vi "HandlePostRequest.vi"(12 "LabVIEW Web Service Request":refnum<class "Web Request.lvclass">) -> (1 "Open %":dbl, 2 "Status":string, 13 "Message":string)   [LabVIEW 2024]
uses:
  <vilib>/wsapi/Web Request.lvclass
  D/Global.vi
  <vilib>/Instr/_visa.llb/VISA Configure Serial Port (Instr).vi
panel:
  out "usb out 2":string
  out "usb out":string
  # "Use the Web Service Request input terminal to call the VIs on the Web Services palette. Do not remove it from the connector pane unless you don't need access to the palette."
  # "Each additional control wired to the connector pane will be available as an input in the URL. To include an indicator in terminal-mode output (the default setting), it must also be wired to the connector pane."
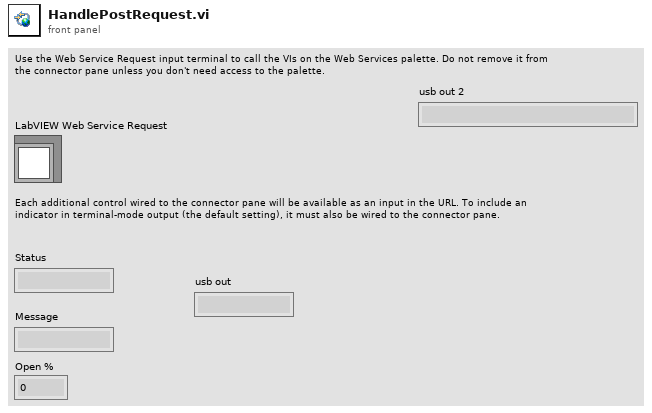
[diagram p1: front panel]
types:
  T1 = cluster{"mode":string, "value":dbl, "t_open":dbl, "t_close":dbl}
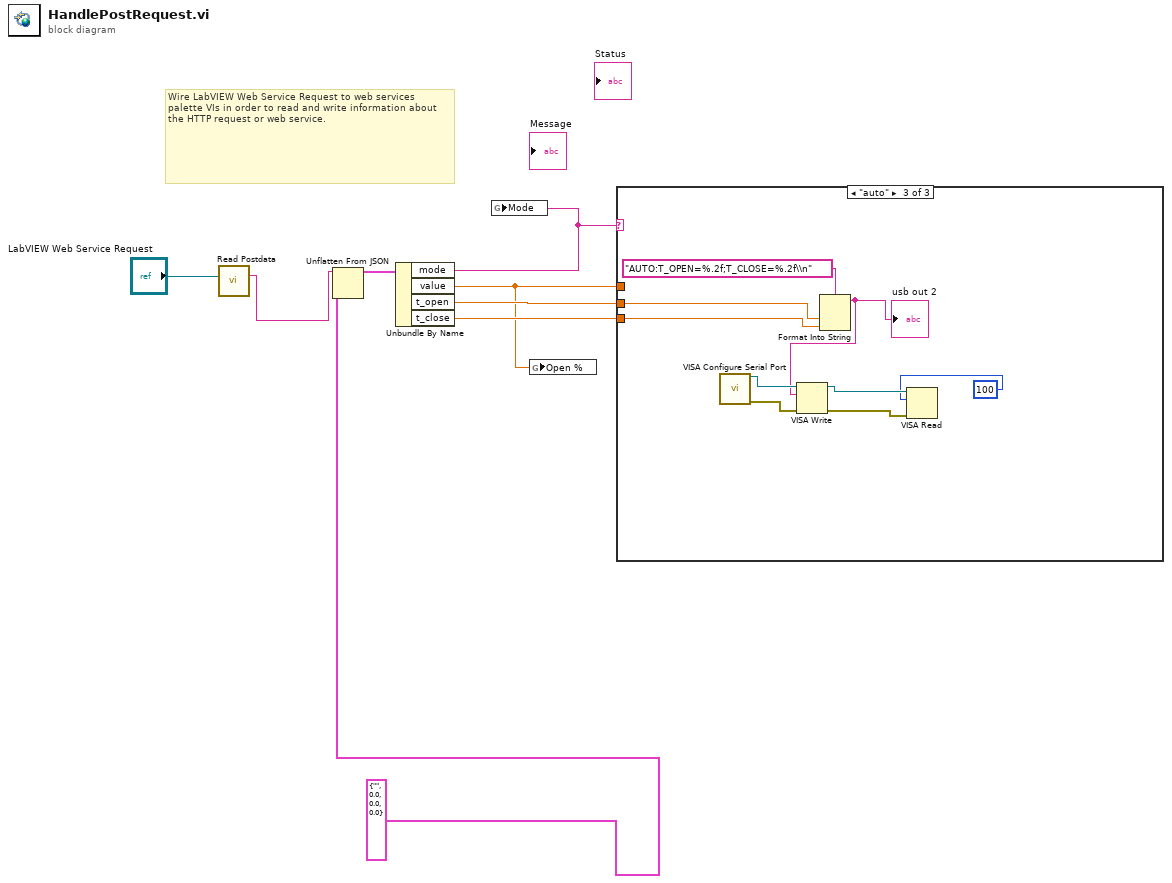
[diagram p0: block diagram]
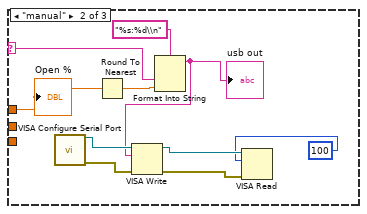
[diagram p3: hidden frame]
diagram:
  # "Wire LabVIEW Web Service Request to web services palette VIs in order to read and write information about the HTTP request or web service."
  n1 = call <vilib>:"Read Postdata.vi"("LabVIEW Web Service Request"="LabVIEW Web Service Request") -> ("postdata"=w7:string)  [unwired: 12 in, 2 out]
  n2 = Unflatten From JSON(JSON string=w7, type and defaults=T1 {"mode"="", "value"=0.0, "t_open"=0.0, "t_close"=0.0} ("Cluster")) -> (value=w6:T1)  [unwired: 5 in, 1 out]
  n3 = Unbundle By Name "Unbundle By Name"(w6) -> ("mode"=w2:string, "value"=w1:dbl, "t_open"=w5:dbl, "t_close"=w4:dbl)
  n4 = global write "Global.vi" "Mode"(w2) -> ()
  n5 = global write "Global.vi" "Open %"(w1) -> ()
  n6 = case shown="\"auto\"" w2 {
    selector: w2 -> [_ w13 _]
    tunnel: w1 -> [_ w12 _]
    tunnel: w5 -> [_ _ w20]
    tunnel: w4 -> [_ _ w19]
    frame "False", Default {
    }
    frame "manual" {
      n7 = call-poly "VISA Configure Serial Port"() -> ("VISA resource name out"=w17:refnum<visa-resource-name>, "error out"=w18:errorcluster)  [unwired: 14 in]
      n8 = Round To Nearest(number=w12) -> (nearest integer value=w11:dbl)
      n9 = Format Into String(format string="%s:%d\\n", w13, w11) -> (resulting string=w10:string)  [unwired: 2 in, 1 out]
      "usb out" <- w10
      n10 = VISA Write(VISA resource name=w17, write buffer=w10, error in (no error)=w18) -> (VISA resource name out=w15:refnum<visa-resource-name>, error out=w16:errorcluster)  [unwired: 1 out]
      n11 = VISA Read(VISA resource name=w15, byte count=100, error in (no error)=w16) -> ()  [unwired: 4 out]
      "Open %" <- w12
    }
    frame "auto" {
      n12 = call-poly "VISA Configure Serial Port"() -> ("VISA resource name out"=w26:refnum<visa-resource-name>, "error out"=w27:errorcluster)  [unwired: 14 in]
      n13 = Format Into String(format string="AUTO:T_OPEN=%.2f;T_CLOSE=%.2f\\n", w20, w19) -> (resulting string=w22:string)  [unwired: 2 in, 1 out]
      "usb out 2" <- w22
      n14 = VISA Write(VISA resource name=w26, write buffer=w22, error in (no error)=w27) -> (VISA resource name out=w24:refnum<visa-resource-name>, error out=w25:errorcluster)  [unwired: 1 out]
      n15 = VISA Read(VISA resource name=w24, byte count=100, error in (no error)=w25) -> ()  [unwired: 4 out]
    }
  }
